vi "ScanFeedback.vi"(2 "measurement type":T1(tab)) -> (1 "V breakdown":dbl, 5 "V depletion":dbl, 6 "Maximum current fluctuations":dbl, 7 "Fraction of good strips":dbl, 8 "Ris [MOhm]":dbl, 9 "Cis [pF/cm]":dbl)   [LabVIEW 2018]
uses:
  <vilib>/Analysis/NI_AALPro.lvlib
  <vilib>/Analysis/NI_AALBase.lvlib
panel:
  out "MEAN":dbl
  out "STD":dbl
  out "Index lin fit 1":dbl
  out "Slope":dbl
  out "capSquare1":dbl[](array[numeric])
  out "volts1":dbl[](array[numeric])
  out "volts2":dbl[](array[numeric])
  out "capSquare2":dbl[](array[numeric])
  out "deriv":dbl[](array[numeric])
  out "Slope 2":dbl
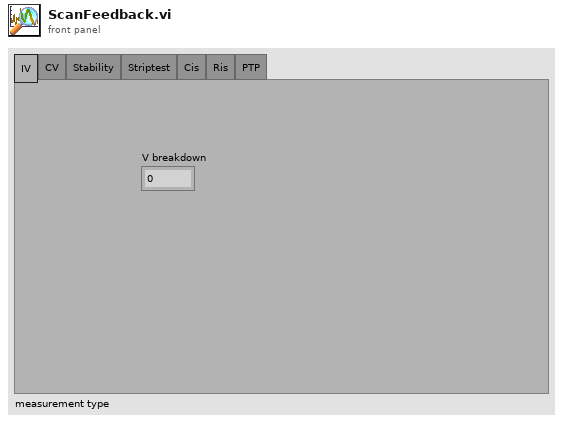
[diagram p1: front panel]
types:
  T1 = enum32{"IV", "CV", "Stability", "Striptest", "Cis", "Ris", "PTP"}
  T2 = enum16{"Reset", "Read Array", "Read Element", "Write Element", "Write Array", "Add Element", "Add Array"}
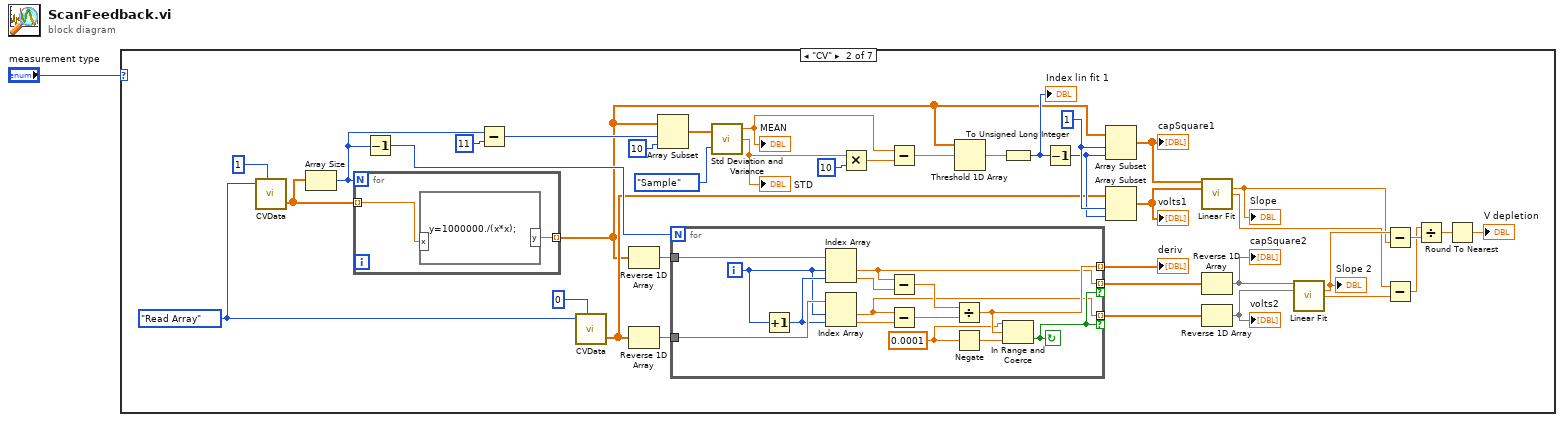
[diagram p0: block diagram]
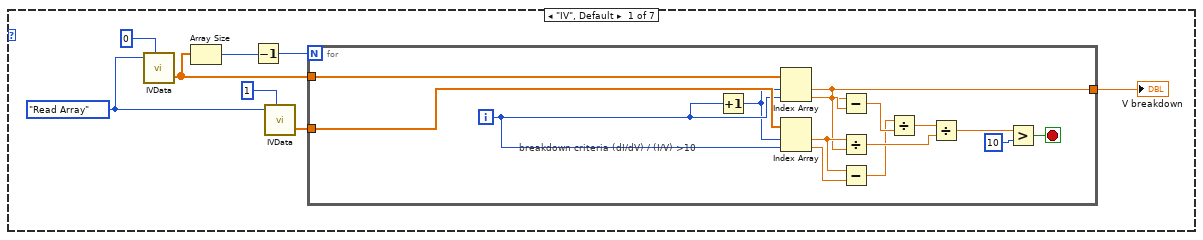
[diagram p2: hidden frame]
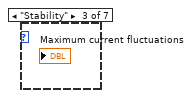
[diagram p3: hidden frame]
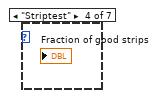
[diagram p4: hidden frame]
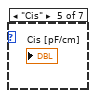
[diagram p5: hidden frame]
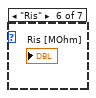
[diagram p6: hidden frame]
diagram:
  n1 = case shown="\"CV\"" "measurement type" {
    frame "IV", Default {
      w7 = T2."Read Array" ("Action")
      n2 = call "IVData.vi"("Action"=w7, "Array No."=0) -> ("Array OUT"=w5:dbl[])  [unwired: 3 in, 1 out]
      n3 = Array Size(array=w5) -> (size(s)=w4:i32)
      n4 = Decrement(x=w4) -> (x-1=w3:i32)
      n5 = call "IVData.vi"("Action"=w7, "Array No."=1) -> ("Array OUT"=w6:dbl[])  [unwired: 3 in, 1 out]
      n6 = for {
        N: w3 -> [_]
        tunnel: w5 -> [w23]
        tunnel: w6 -> [w24]
        tunnel: [w10] -> w2
        i -> [w20]
        stop <- w11 stop-if-true
        # "breakdown criteria (dI/dV) / (I/V) >10"
        n7 = Increment(x=w20) -> (x+1=w19:i32)
        n8 = Index Array(array=w23, index #1=w19, index #2=w20) -> (element #1=w10:dbl, element #2=w22:dbl)
        n9 = Index Array(array=w24, index #1=w19, index #2=w20) -> (element #1=w14:dbl, element #2=w21:dbl)
        n10 = Subtract(x=w10, y=w22) -> (x-y=w16:dbl)
        n11 = Divide(x=w14, y=w10) -> (x/y=w17:dbl)
        n12 = Subtract(x=w14, y=w21) -> (x-y=w15:dbl)
        n13 = Divide(x=w15, y=w16) -> (x/y=w18:dbl)
        n14 = Divide(x=w18, y=w17) -> (x/y=w12:dbl)
        n15 = Greater?(x=w12, y=10) -> (0:w11:bool)
      }
      "V breakdown" <- w2
    }
    frame "CV" {
      w35 = T2."Read Array" ("Action")
      w32 = 1
      n16 = call "CVData.vi"("Action"=w35, "Array No."=1) -> ("Array OUT"=w26:dbl[])  [unwired: 3 in, 1 out]
      n17 = Array Size(array=w26) -> (size(s)=w27:i32)
      n18 = for {
        N: w27 -> [_]
        tunnel: w26 -> [w65] mode=indexing
        tunnel: [w64] -> w25 mode=indexing
        n19 = formula code="y=1000000./(x*x);"("x"=w65) -> ("y"=w64:dbl)
      }
      n20 = Decrement(x=w27) -> (x-1=w48:i32)
      n21 = Subtract(x=w27, y=11) -> (x-y=w62:i32)
      n22 = call "CVData.vi"("Action"=w35, "Array No."=0) -> ("Array OUT"=w29:dbl[])  [unwired: 3 in, 1 out]
      n23 = Reverse 1D Array(array=w25) -> (reversed array=w51:dbl[])
      n24 = Reverse 1D Array(array=w29) -> (reversed array=w28:dbl[])
      n25 = Array Subset(array=w25, index=w62, length=10) -> (w60:dbl[])
      n26 = for {
        N: w48 -> [_]
        tunnel: w51 -> [w79]
        tunnel: [w72] -> w50 mode=indexing if=w73
        tunnel: [w68] -> w47 mode=indexing if=w73
        tunnel: [w76] -> w44 mode=indexing
        tunnel: w28 -> [w71]
        i -> [w69]
        stop <- w73 continue-if-true
        w74 = 0.0001
        n27 = Increment(x=w69) -> (x+1=w70:i32)
        n28 = Index Array(array=w79, index #1=w69, index #2=w70) -> (element #1=w72:dbl, element #2=w77:dbl)
        n29 = Index Array(array=w71, index #1=w69, index #2=w70) -> (element #1=w68:dbl, element #2=w67:dbl)
        n30 = Subtract(x=w72, y=w77) -> (x-y=w78:dbl)
        n31 = Subtract(x=w68, y=w67) -> (x-y=w66:dbl)
        n32 = Divide(x=w78, y=w66) -> (x/y=w76:dbl)
        n33 = Negate(x=w74) -> (-x=w75:dbl)
        n34 = In Range and Coerce(upper limit=w74, x=w76, lower limit=w75) -> (In Range?=w73:bool)  [unwired: 1 out]
      }
      "deriv" <- w44
      n35 = call <vilib>:"Std Deviation and Variance.vi"("X"=w60, "Weighting (Sample)"=enum16{"Sample", "Population"}."Sample") -> ("mean"=w56:dbl, "standard deviation"=w45:dbl)  [unwired: 1 out]
      "MEAN" <- w56
      "STD" <- w45
      n36 = Multiply(x=w45, y=10) -> (x*y=w57:dbl)
      n37 = Subtract(x=w56, y=w57) -> (x-y=w55:dbl)
      n38 = Threshold 1D Array(2:w55, 3:w25) -> (0:w54:dbl)  [unwired: 1 in]
      n39 = To Unsigned Long Integer(number=w54) -> (unsigned 32bit integer=w53:u32)
      "Index lin fit 1" <- w53
      n40 = Decrement(x=w53) -> (x-1=w31:u32)
      n41 = Array Subset(array=w25, index=w32, length=w31) -> (w52:dbl[])
      "capSquare1" <- w52
      n42 = Array Subset(array=w29, index=w32, length=w31) -> (w30:dbl[])
      "volts1" <- w30
      n43 = call <vilib>:"Linear Fit.vi"("Y"=w52, "X"=w30) -> ("slope"=w42:dbl, "intercept"=w40:dbl)  [unwired: 9 in, 3 out]
      "Slope" <- w42
      n44 = Reverse 1D Array(array=w50) -> (reversed array=w49:dbl[])
      "capSquare2" <- w49
      n45 = Reverse 1D Array(array=w47) -> (reversed array=w46:dbl[])
      "volts2" <- w46
      n46 = call <vilib>:"Linear Fit.vi"("Y"=w49, "X"=w46) -> ("slope"=w43:dbl, "intercept"=w41:dbl)  [unwired: 9 in, 3 out]
      "Slope 2" <- w43
      n47 = Subtract(x=w43, y=w42) -> (x-y=w39:dbl)
      n48 = Subtract(x=w40, y=w41) -> (x-y=w38:dbl)
      n49 = Divide(x=w38, y=w39) -> (x/y=w37:dbl)
      n50 = Round To Nearest(number=w37) -> (nearest integer value=→"V depletion":dbl)
    }
    frame "Stability" {
    }
    frame "Striptest" {
    }
    frame "Cis" {
    }
    frame "Ris" {
    }
    frame "PTP" {
    }
  }
